vi "get_DTA_fileConfig.vi"(8 "Error In":errorcluster, 11 "FGV_data":T1) -> (0 "Error Out":errorcluster, 3 "FGV_data out":T1)   [LabVIEW 2018]
uses:
  FGV/FGV_data.ctl
  config_data.ctl
  <vilib>/Utility/miscctls.llb/LVDateTimeRec.ctl
panel:
  out "IDs":u8[](array[numeric])
  out "data":u8[][](array[numeric])
  out "Array":u8[](array[numeric])
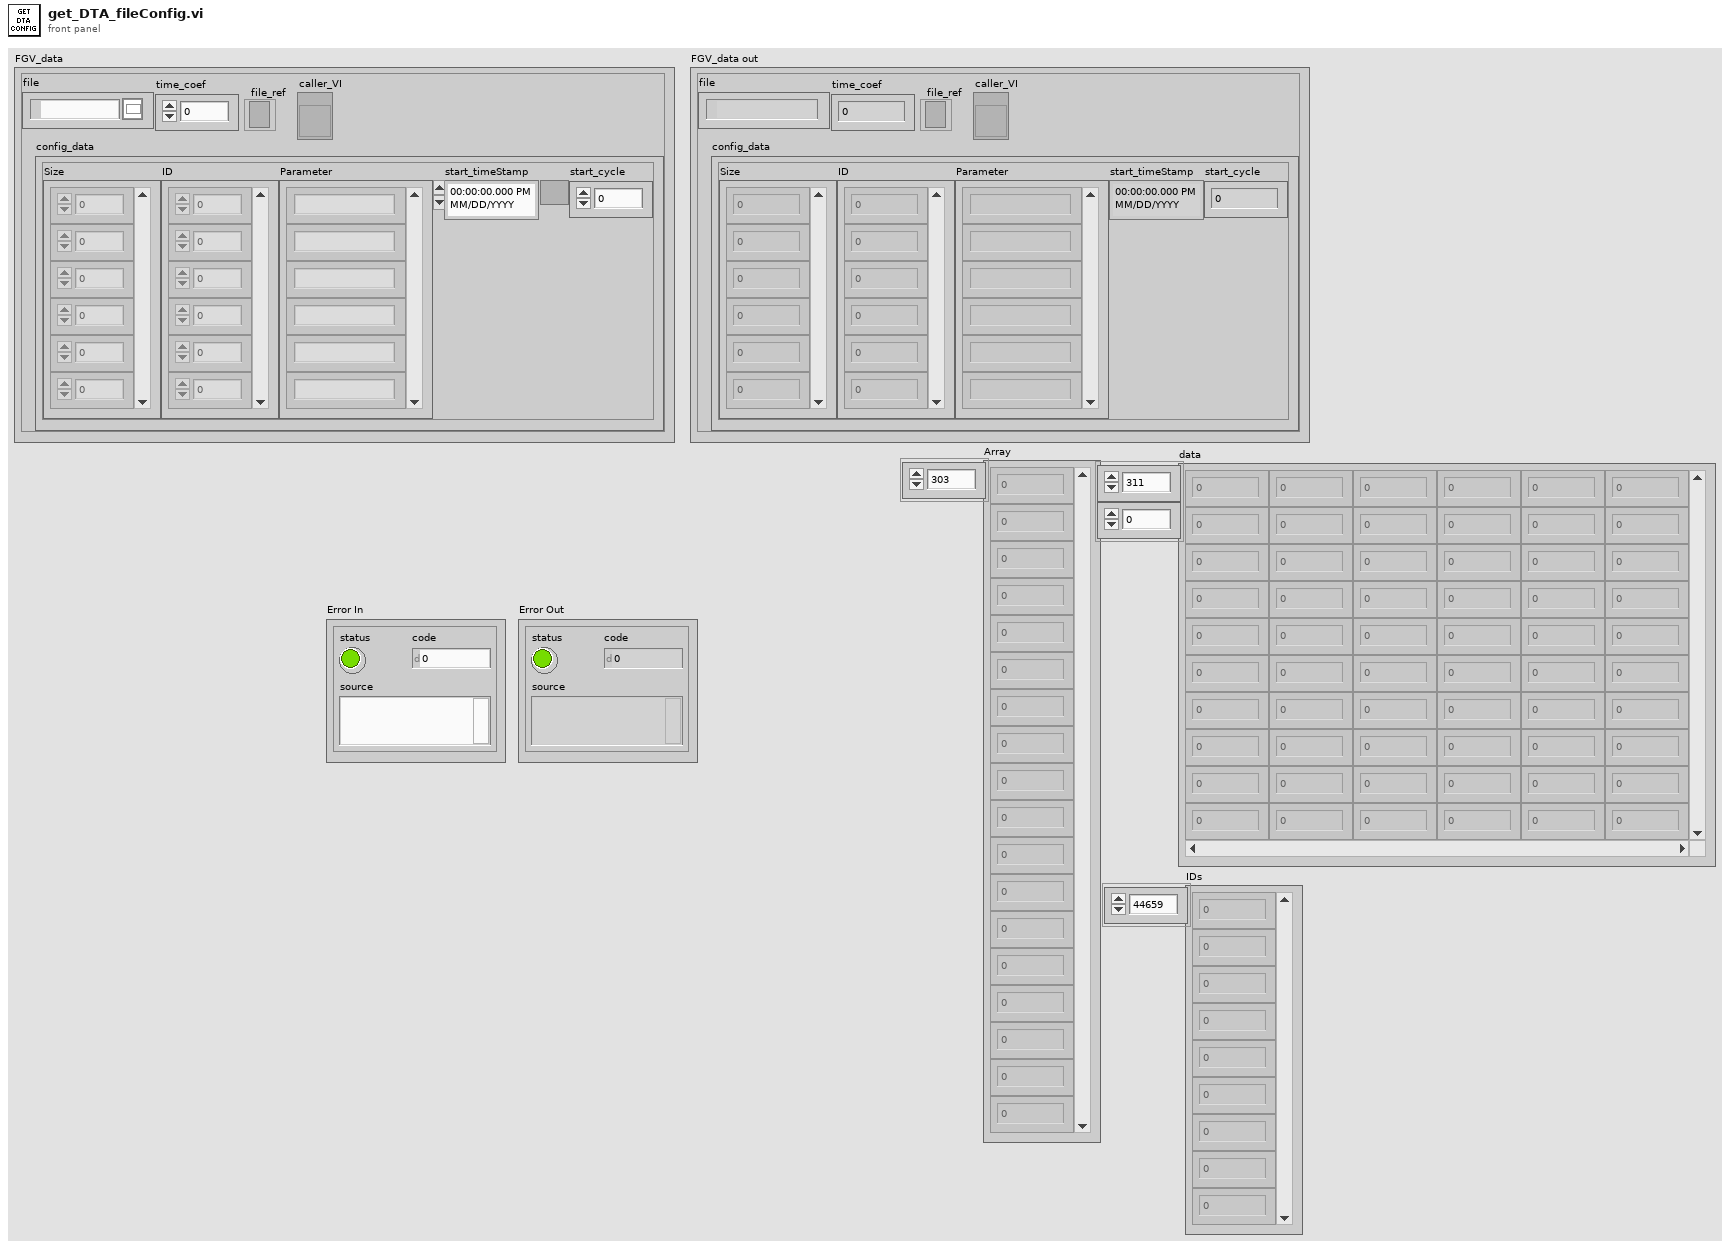
[diagram p1: front panel]
types:
  T1 = typedef "FGV_data.ctl" = cluster{"file":path, "time_coef":dbl, "config_data":T2, "file_ref":refnum<file>, "caller_VI":refnum<vi>}
  T2 = typedef "config_data.ctl" = cluster{"Size":i32[], "ID":u8[], "Parameter":string[], "start_timeStamp":timestamp, "start_cycle":u64}
  T3 = typedef "LVDateTimeRec.ctl" = cluster{"fractional second":dbl, "second":i32, "minute":i32, "hour":i32, "day of month":i32, "month":i32, "year":i32, "day of week":i32, "day of year":i32, "DST":i32}
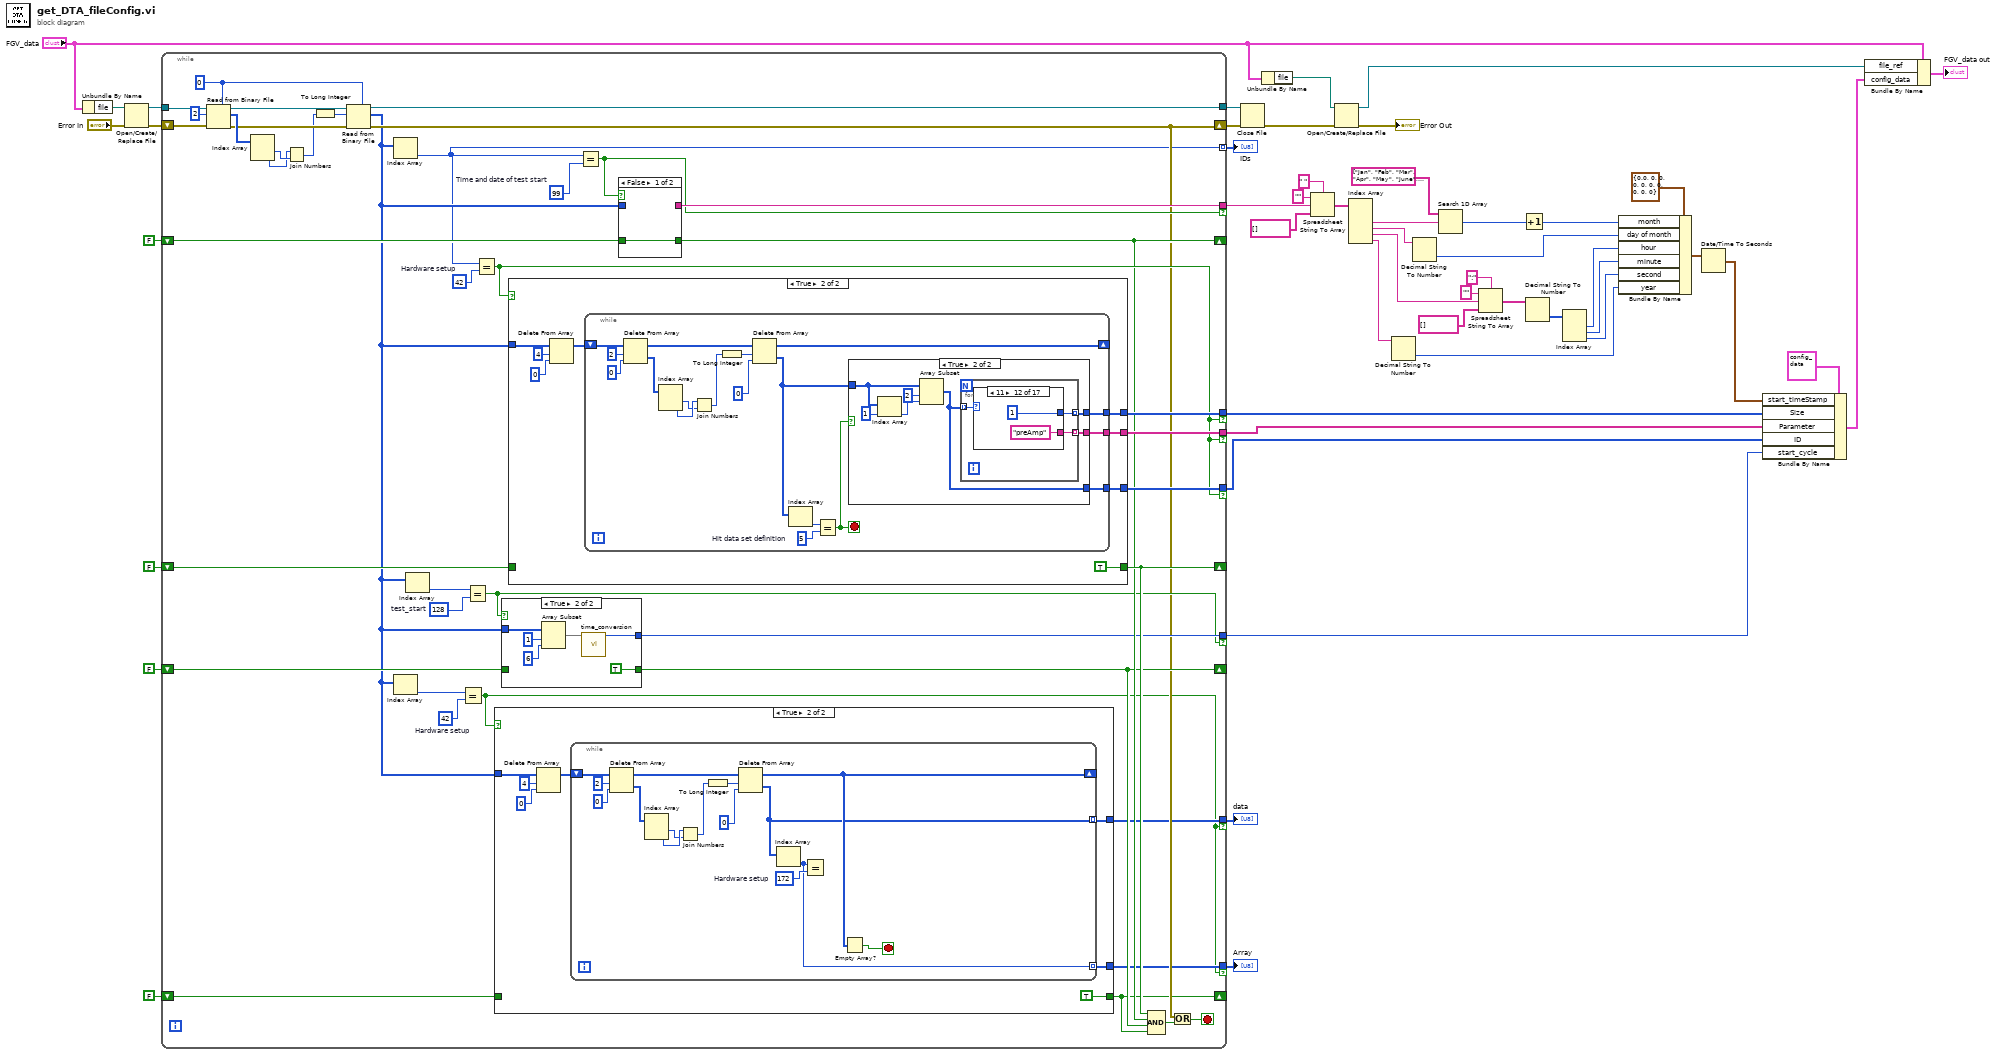
[diagram p0: block diagram]
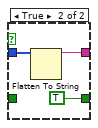
[diagram p3: hidden frame]
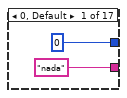
[diagram p6: hidden frame]
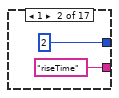
[diagram p7: hidden frame]
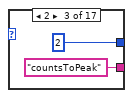
[diagram p8: hidden frame]
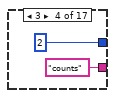
[diagram p9: hidden frame]
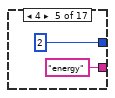
[diagram p10: hidden frame]
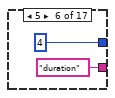
[diagram p11: hidden frame]
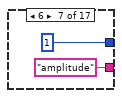
[diagram p12: hidden frame]
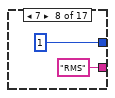
[diagram p13: hidden frame]
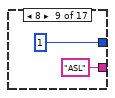
[diagram p14: hidden frame]
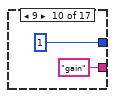
[diagram p15: hidden frame]
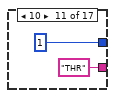
[diagram p16: hidden frame]
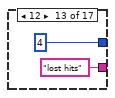
[diagram p17: hidden frame]
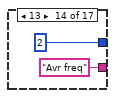
[diagram p18: hidden frame]
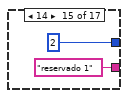
[diagram p19: hidden frame]
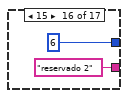
[diagram p20: hidden frame]
diagram:
  n1 = Unbundle By Name("FGV_data") -> ("file"=w48:path)
  n2 = Open/Create/Replace File(file path (use dialog)=w48, error in="Error In") -> (refnum out=w50:refnum<file>, error out=w49:errorcluster)  [unwired: 4 in, 1 out]
  n3 = while {
    tunnel: w50 -> [w92]
    shift-right: [w60] -> w13
    shift-left: w49 -> [w84]
    tunnel: [w81] -> w40 if=w80
    tunnel: [w77] -> w43 if=w74
    tunnel: [w76] -> w42 if=w74
    tunnel: [w75] -> w41 if=w74
    shift-right: [w71] -> _
    shift-left: FALSE -> [w73]
    shift-right: [w70] -> _
    shift-left: FALSE -> [w72]
    tunnel: [w69] -> w12
    shift-right: [w65] -> _
    shift-left: FALSE -> [w66]
    tunnel: [w64] -> w5 if=w63
    shift-right: [w54] -> _
    shift-left: FALSE -> [w56]
    tunnel: [w55] -> w3 if=w52
    tunnel: [w53] -> w2 if=w52
    tunnel: [w51] -> w1 mode=indexing
    stop <- w61 stop-if-true
    w59 = u8 42  # Hardware setup
    w67 = u8 128  # test_start
    w78 = u8 42  # Hardware setup
    w82 = u8 99  # Time and date of test start
    w87 = u8 0
    n4 = Read from Binary File(5:w87, 8:w84, 10:2 ("count (1)"), 11:w92) -> (0:w88:errorcluster, 2:w90:u8[], 3:w89:refnum<file>)  [unwired: 2 in, 1 out]
    n5 = Index Array(array=w90) -> (element #1=w86:u8, element #2=w85:u8)  [unwired: 2 in]
    n6 = Join Numbers(hi=w85, lo=w86) -> ((hi.lo)=w83:u16)
    n7 = To Long Integer(number=w83) -> (32bit integer=w79:i32)
    n8 = Read from Binary File(5:w87, 8:w88, 10:w79, 11:w89) -> (0:w60:errorcluster, 2:w57:u8[], 3:w69:refnum<file>)  [unwired: 2 in, 1 out]
    n9 = Index Array(array=w57) -> (element=w51:u8)  [unwired: 1 in]
    n10 = Index Array(array=w57) -> (element=w58:u8)  [unwired: 1 in]
    n11 = Index Array(array=w57) -> (element=w68:u8)  [unwired: 1 in]
    n12 = Equal?(x=w58, y=w59) -> (x = y?=w52:bool)
    n13 = Equal?(x=w68, y=w67) -> (x = y?=w63:bool)
    n14 = Equal?(x=w51, y=w78) -> (x = y?=w74:bool)
    n15 = case shown="True" w52 {
      tunnel: w57 -> [_ w180]
      tunnel: [w175 TRUE] -> w54
      tunnel: w56 -> [w175 _]
      tunnel: [_ w177] -> w55
      tunnel: [_ w176] -> w53
      frame False {
      }
      frame True {
        n16 = Delete From Array(array=w180, length=4, index=0) -> (array with subset deleted=w181:u8[])  [unwired: 1 out]
        n17 = while {
          shift-right: [w185] -> _
          shift-left: w181 -> [w197]
          tunnel: [w184] -> w177 mode=indexing
          tunnel: [w183] -> w176 mode=indexing
          stop <- w186 stop-if-true
          w187 = u8 172  # Hardware setup
          n18 = Delete From Array(array=w197, length=2, index=0) -> (deleted portion=w190:u8[], array with subset deleted=w195:u8[])
          n19 = Index Array(array=w190) -> (element #1=w191:u8, element #2=w192:u8)  [unwired: 2 in]
          n20 = Join Numbers(hi=w192, lo=w191) -> ((hi.lo)=w189:u16)
          n21 = To Long Integer(number=w189) -> (32bit integer=w188:i32)
          n22 = Delete From Array(array=w195, length=w188, index=0) -> (deleted portion=w183:u8[], array with subset deleted=w185:u8[])
          n23 = Index Array(array=w183) -> (element=w184:u8)  [unwired: 1 in]
          n24 = Equal?(x=w184, y=w187) -> ()  [unwired: 1 out]
          n25 = Empty Array?(array=w185) -> (empty?=w186:bool)
        }
      }
    }
    n26 = case shown="True" w63 {
      tunnel: w57 -> [_ w97]
      tunnel: [_ w94] -> w64
      tunnel: [w93 TRUE] -> w65
      tunnel: w66 -> [w93 _]
      frame False {
      }
      frame True {
        n27 = Array Subset(array=w97, index=1, length=6) -> (w95:u8[])
        n28 = call "time_conversion.vi"("array_time"=w95) -> ("time_U64"=w94:u64)  [unwired: 10 in]
      }
    }
    n29 = case shown="True" w74 {
      tunnel: w57 -> [_ w110]
      tunnel: [_ w108] -> w77
      tunnel: [_ w107] -> w76
      tunnel: [_ w106] -> w75
      tunnel: [w104 TRUE] -> w71
      tunnel: w73 -> [w104 _]
      frame False {
      }
      frame True {
        n30 = Delete From Array(array=w110, length=4, index=0) -> (array with subset deleted=w111:u8[])  [unwired: 1 out]
        n31 = while {
          shift-right: [w127] -> _
          shift-left: w111 -> [w130]
          tunnel: [w115] -> w108
          tunnel: [w114] -> w107
          tunnel: [w113] -> w106
          stop <- w117 stop-if-true
          w118 = u8 5  # Hit data set definition
          n32 = Delete From Array(array=w130, length=2, index=0) -> (deleted portion=w122:u8[], array with subset deleted=w128:u8[])
          n33 = Index Array(array=w122) -> (element #1=w123:u8, element #2=w124:u8)  [unwired: 2 in]
          n34 = Join Numbers(hi=w124, lo=w123) -> ((hi.lo)=w121:u16)
          n35 = To Long Integer(number=w121) -> (32bit integer=w120:i32)
          n36 = Delete From Array(array=w128, length=w120, index=0) -> (deleted portion=w116:u8[], array with subset deleted=w127:u8[])
          n37 = Index Array(array=w116) -> (element=w119:u8)  [unwired: 1 in]
          n38 = Equal?(x=w119, y=w118) -> (x = y?=w117:bool)
          n39 = case shown="True" w117 {
            tunnel: w116 -> [_ w136]
            tunnel: [_ w133] -> w115
            tunnel: [_ w132] -> w114
            tunnel: [_ w131] -> w113
            frame False {
            }
            frame True {
              n40 = Index Array(array=w136, index=1) -> (element=w135:u8)
              n41 = Array Subset(array=w136, index=2, length=w135) -> (w131:u8[])
              n42 = for {
                tunnel: w131 -> [w140] mode=indexing
                tunnel: [w139] -> w133 mode=indexing
                tunnel: [w138] -> w132 mode=indexing
                n43 = case shown="11" w140 {
                  tunnel: [0 ("length") 2 ("length") 2 ("length") 2 ("length") 2 ("length") 4 ("length") 1 ("length") 1 ("length") 1 ("length") 1 ("length") 1 ("length") 1 ("length") 4 ("length") 2 ("length") 2 ("length") 6 ("length") 4 ("length")] -> w139
                  tunnel: ["nada" "riseTime" "countsToPeak" "counts" "energy" "duration" "amplitude" "RMS" "ASL" "gain" "THR" "preAmp" "lost hits" "Avr freq" "reservado 1" "reservado 2" "reservado 3"] -> w138
                  frame 0, Default {
                  }
                  frame 1 {
                  }
                  frame 2 {
                  }
                  frame 3 {
                  }
                  frame 4 {
                  }
                  frame 5 {
                  }
                  frame 6 {
                  }
                  frame 7 {
                  }
                  frame 8 {
                  }
                  frame 9 {
                  }
                  frame 10 {
                  }
                  frame 11 {
                  }
                  frame 12 {
                  }
                  frame 13 {
                  }
                  frame 14 {
                  }
                  frame 15 {
                  }
                  frame 16 {
                  }
                }
              }
            }
          }
        }
      }
    }
    n44 = Equal?(x=w51, y=w82) -> (x = y?=w80:bool)
    n45 = case shown="False" w80 {
      tunnel: w57 -> [_ w103]
      tunnel: [_ w102] -> w81
      tunnel: [w100 TRUE] -> w70
      tunnel: w72 -> [w100 _]
      frame False {
      }
      frame True {
        n46 = Flatten To String(anything=w103) -> (data string=w102:string)  [unwired: 3 in, 2 out]
      }
    }
    n47 = Compound Arithmetic op=AND(w71, w70, w65, w54) -> (w62:bool)
    n48 = Or(x=w60, y=w62) -> (x .or. y?=w61:bool)
  }
  "Array" <- w3
  "data" <- w2
  "IDs" <- w1
  n49 = Close File(refnum=w12, error in=w13) -> (error out=w11:errorcluster)  [unwired: 1 out]
  n50 = Unbundle By Name("FGV_data") -> ("file"=w9:path)
  n51 = Spreadsheet String To Array(delimiter (Tab)=" ", format string="", spreadsheet string=w40, array type (2D Dbl)=string[] []) -> (array=w36:string[])
  n52 = Open/Create/Replace File(file path (use dialog)=w9, error in=w11) -> (refnum out=w7:refnum<file>, error out=→"Error Out":errorcluster)  [unwired: 4 in, 1 out]
  n53 = Index Array(array=w36) -> (element #2=w33:string, element #3=w30:string, element #4=w25:string, element #5=w19:string)  [unwired: 5 in, 1 out]
  n54 = Decimal String To Number(string=w19) -> (number=w18:i32)  [unwired: 2 in, 1 out]
  n55 = Decimal String To Number(string=w30) -> (number=w29:i32)  [unwired: 2 in, 1 out]
  n56 = Search 1D Array(1D array=string[] ["Jan", "Feb", "Mar", "Apr", "May", "June", "July", "Aug", "Sept", "Oct", "Nov", "Dec"], element=w33) -> (index of element=w32:i32)  [unwired: 1 in]
  n57 = Spreadsheet String To Array(delimiter (Tab)=":", format string="", spreadsheet string=w25, array type (2D Dbl)=string[] []) -> (array=w24:string[])
  n58 = Increment(x=w32) -> (x+1=w31:i32)
  n59 = Decimal String To Number(string=w24) -> (number=w23:i32[])  [unwired: 2 in, 1 out]
  n60 = Index Array(array=w23) -> (element #1=w22:i32, element #2=w21:i32, element #3=w20:i32)  [unwired: 3 in]
  n61 = Bundle By Name(cluster=T3 {"fractional second"=0.0, "second"=0, "minute"=0, "hour"=0, "day of month"=0, "month"=0, "year"=0, "day of week"=0, "day of year"=0, "DST"=0} ("date time rec"), "month"=w31, "day of month"=w29, "hour"=w22, "minute"=w21, "second"=w20, "year"=w18) -> (w17:T3)
  n62 = Date/Time To Seconds(2:w17) -> (0:w16:timestamp)  [unwired: 1 in]
  n63 = Bundle By Name(cluster=T2 {"Size"=[2, 2, 2, 2, 4, 1, 1, 1, 2, 0, 0, 0, 0, 0], "ID"=[2, 2, 2, 2, 4, 1, 1, 1, 2, 0, 0, 0, 0, 0], "Parameter"=[], "start_timeStamp"=timestamp(0 s since 1904-01-01), "start_cycle"=0} ("config_data"), "start_timeStamp"=w16, "Size"=w43, "Parameter"=w42, "ID"=w41, "start_cycle"=w5) -> (w15:T2)
  n64 = Bundle By Name(cluster="FGV_data", "file_ref"=w7, "config_data"=w15) -> (→"FGV_data out":T1)
